vi "sendCmdFromTcpClient.vi"(6 "timeout ms (1000)":i32=1000, 8 "error in (no error)":errorcluster, 9 "sequence_id":i32[](array[numeric])=[0, 1], 10 "commands":string[](array[string])=["move", "stop"], 11 "connectionID":refnum<k5>) -> (0 "error out":errorcluster, 2 "ack received":string[](array[string]), 3 "connectionID":refnum<k5>)   [LabVIEW 2018]
doc: "Generate commands as JSON packets and send them to TCP server, and then read the response from TCP server."
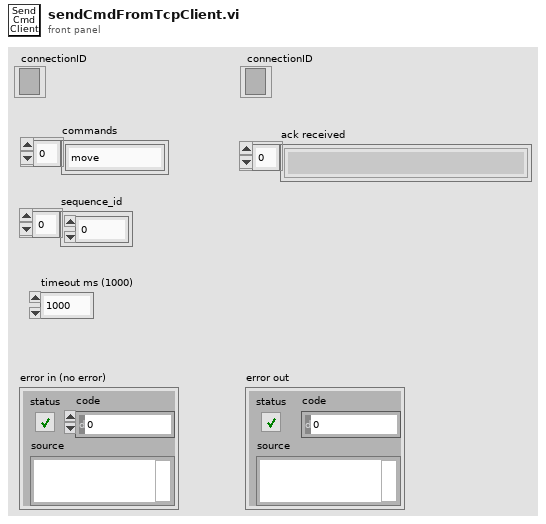
[diagram p1: front panel]
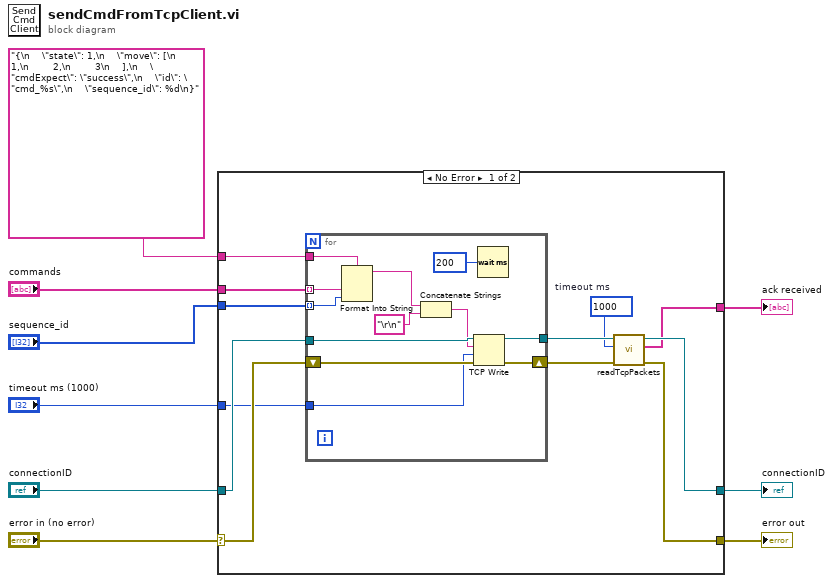
[diagram p0: block diagram]
diagram:
  n1 = case shown="No Error" "error in (no error)" {
    selector: "error in (no error)" -> [w12 w35]
    tunnel: [w16 w34] -> w9
    tunnel: [w15 w35] -> w7
    tunnel: [w14 _] -> w6
    tunnel: "connectionID" -> [w21 w34]
    tunnel: "{\n    \"state\": 1,\n    \"move\": [\n        1,\n        2,\n        3\n    ],\n    \"cmdExpect\": \"success\",\n    \"id\": \"cmd_%s\",\n    \"sequence_id\": %d\n}" ("Display") -> [w13 _]
    tunnel: "commands" -> [w20 _]
    tunnel: "sequence_id" -> [w19 _]
    tunnel: "timeout ms (1000)" -> [w11 _]
    frame No Error {
      w10 = 1000  # timeout ms
      n2 = for {
        shift-right: [w32] -> w17
        shift-left: w12 -> [w28]
        tunnel: w13 -> [w26]
        tunnel: w20 -> [w25] mode=indexing
        tunnel: w19 -> [w24] mode=indexing
        tunnel: w21 -> [w29]
        tunnel: [w30] -> w18
        tunnel: w11 -> [w22]
        n3 = Format Into String(format string=w26, w25, w24) -> (resulting string=w23:string)  [unwired: 2 in, 1 out]
        n4 = Concatenate Strings(w23, "\r\n" ("string")) -> (w27:string)
        n5 = TCP Write(connection ID=w29, data in=w27, error in (no error)=w28, 9:w22) -> (connection ID out=w30:refnum<k5>, error out=w32:errorcluster)  [unwired: 1 out]
        n6 = Wait (ms)(milliseconds to wait=u32 200) -> ()  [unwired: 1 out]
      }
      n7 = call "readTcpPackets.vi"("error in (no error)"=w17, "timeout ms"=w10, "connection ID in"=w18) -> ("error out"=w15:errorcluster, "TCP packets"=w14:string[], "connection ID out"=w16:refnum<k5>)  [unwired: 6 in]
    }
    frame Error {
    }
  }
  "connectionID" <- w9
  "error out" <- w7
  "ack received" <- w6
